vi "_Read_C.vi"(8 "error in (no error)":errorcluster, 11 "Postgres Connector In":refnum<class "Postgres Connector.lvclass">) -> (0 "error out":errorcluster, 1 "Another Query?":bool, 2 "No return?":bool, 3 "Postgres Connector Out":refnum<class "Postgres Connector.lvclass">)   [LabVIEW 2019, in "PG_LIB.lvlib" / "Postgres Connector.lvclass"]
doc: "This VI decode the \"C\" section of the message sent by the database. It also check if a another query has been sent. It return the type of query that has been completed"
uses:
  Postgres Connector.lvclass
  Cluster_Reader_Infos.ctl
  Enum_RowDescription_State_Machine.ctl
  Postgres Connector.lvclass/Postgres Connector.ctl
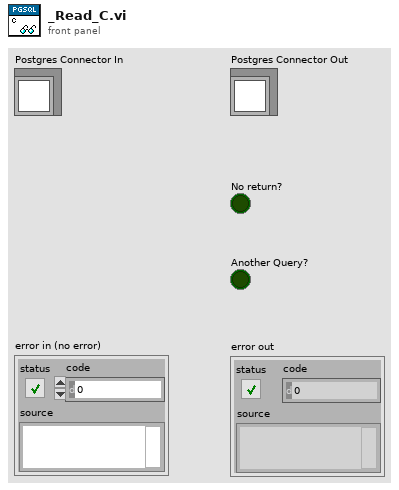
[diagram p1: front panel]
types:
  T1 = typedef "PG_LIB.lvlib/Postgres Connector.lvclass/Cluster_Reader_Infos.ctl" = cluster{"Byte Length":i32}
  T2 = typedef "PG_LIB.lvlib/Postgres Connector.lvclass/Enum_RowDescription_State_Machine.ctl" = enum16{"Check For Error", "Wait For T", "Wait For D", "Wait For Z", "C Byte Length", "Z Byte Length", "n Byte Length", "Byte Length", "Get Infos", "Check For End", "Flush", "Quit"}
  T3 = enum16{"Standard", "Buffered", "CRLF", "Immediate"}
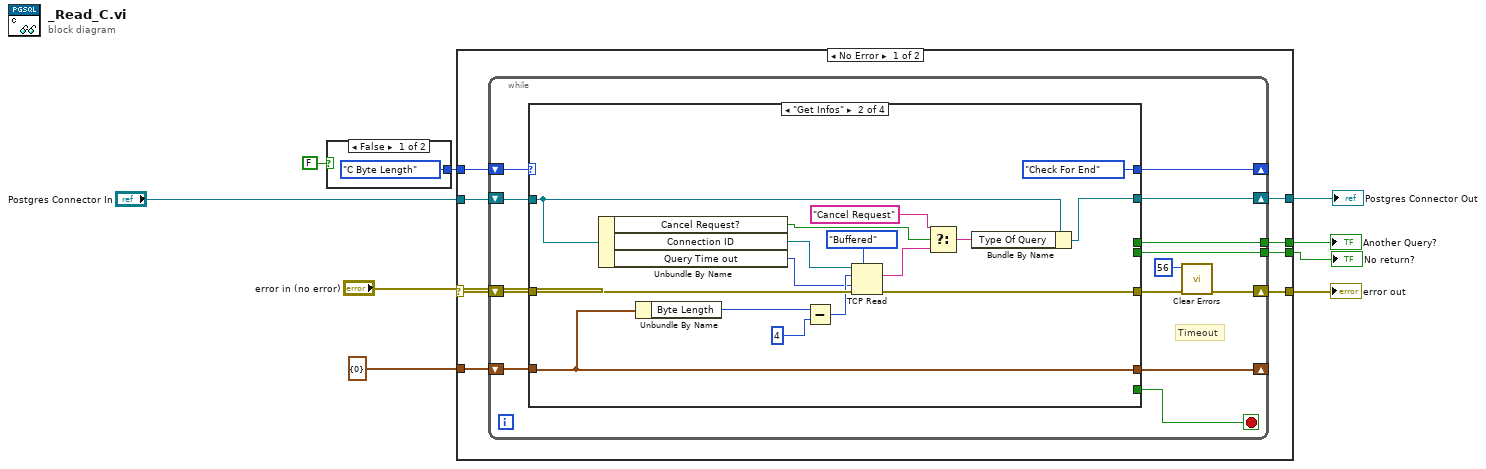
[diagram p0: block diagram]
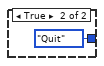
[diagram p2: hidden frame]
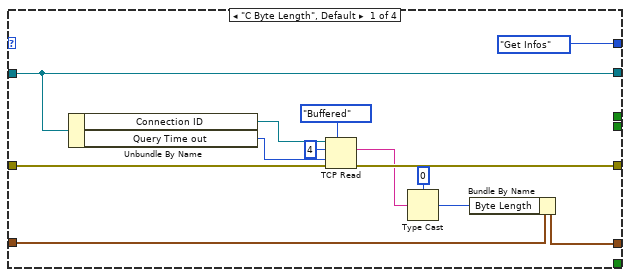
[diagram p3: hidden frame]
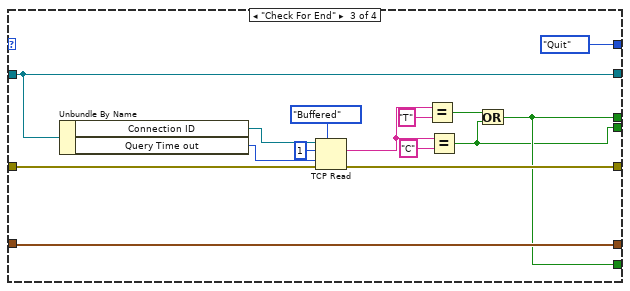
[diagram p4: hidden frame]
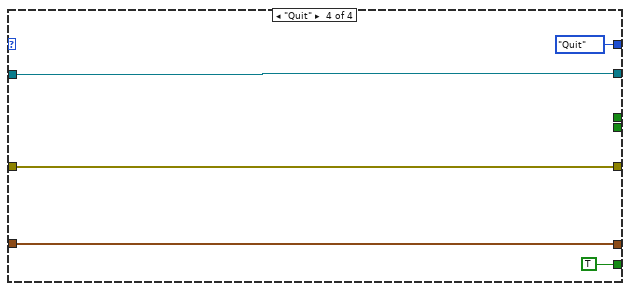
[diagram p5: hidden frame]
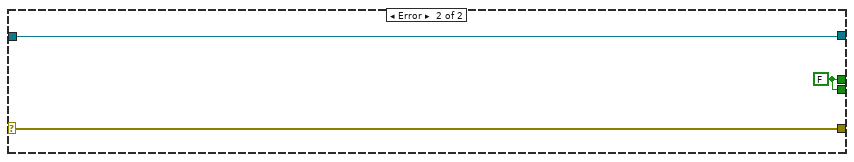
[diagram p6: hidden frame]
diagram:
  n1 = case shown="False" FALSE {
    tunnel: [Enum_RowDescription_State_Machine."C Byte Length" Enum_RowDescription_State_Machine."Quit"] -> w8
    frame False {
    }
    frame True {
    }
  }
  n2 = case shown="No Error" "error in (no error)" {
    selector: "error in (no error)" -> [w18 w84]
    tunnel: "Postgres Connector In" -> [w19 w83]
    tunnel: w8 -> [w17 _]
    tunnel: [w16 w84] -> w7
    tunnel: T1 {"Byte Length"=0} ("Reader_Infos") -> [w15 _]
    tunnel: [w14 w82] -> w5
    tunnel: [w13 w83] -> w4
    tunnel: [w12 w82] -> w3
    frame No Error {
      n3 = while {
        shift-right: [w28] -> w16
        shift-left: w18 -> [w31]
        shift-right: [w26] -> _
        shift-left: w17 -> [w30]
        shift-right: [w24] -> _
        shift-left: w15 -> [w25]
        tunnel: [w22] -> w14
        shift-right: [w21] -> w13
        shift-left: w19 -> [w32]
        tunnel: [w20] -> w12
        stop <- w23 stop-if-true
        # "Timeout"
        n4 = case shown="\"Get Infos\"" w30 {
          tunnel: w32 -> [w41 w52 w68 w77]
          tunnel: w31 -> [w42 w59 w72 w80]
          tunnel: [w40 w58 w71 w80] -> w29
          tunnel: [Enum_RowDescription_State_Machine."Get Infos" Enum_RowDescription_State_Machine."Check For End" Enum_RowDescription_State_Machine."Quit" Enum_RowDescription_State_Machine."Quit"] -> w26
          tunnel: w25 -> [w39 w56 w70 w81]
          tunnel: [w38 w56 w70 w81] -> w24
          tunnel: [_ _ w65 TRUE] -> w23
          tunnel: [_ _ w65 _] -> w22
          tunnel: [w41 w51 w68 w77] -> w21
          tunnel: [_ _ w64 _] -> w20
          frame "C Byte Length", Default {
            n5 = Unbundle By Name(w41) -> ("Connection ID"=w44:refnum<k5>, "Query Time out"=w33:i32)
            n6 = TCP Read(connection ID=w44, bytes to read=4, error in (no error)=w42, 7:T3."Buffered" ("mode (standard)"), 9:w33) -> (data out=w34:string, error out=w40:errorcluster)  [unwired: 1 out]
            n7 = Type Cast(type=0, x=w34) -> (*(type *) &x=w35:i32)
            n8 = Bundle By Name(cluster=w39, "Byte Length"=w35) -> (w38:T1)
          }
          frame "Get Infos" {
            n9 = Unbundle By Name(w52) -> ("Cancel Request?"=w46:bool, "Connection ID"=w60:refnum<k5>, "Query Time out"=w50:i32)
            n10 = Unbundle By Name(w56) -> ("Byte Length"=w55:i32)
            n11 = Subtract(x=w55, y=4 ("bytes to read")) -> (x-y=w54:i32)
            n12 = TCP Read(connection ID=w60, bytes to read=w54, error in (no error)=w59, 7:T3."Buffered" ("mode (standard)"), 9:w50) -> (data out=w49:string, error out=w58:errorcluster)  [unwired: 1 out]
            n13 = Select(t="Cancel Request", s=w46, f=w49) -> (s? t:f=w48:string)
            n14 = Bundle By Name(cluster=w52, "Type Of Query"=w48) -> (w51:refnum<class "Postgres Connector.lvclass">)
          }
          frame "Check For End" {
            n15 = Unbundle By Name(w68) -> ("Connection ID"=w75:refnum<k5>, "Query Time out"=w62:i32)
            n16 = TCP Read(connection ID=w75, bytes to read=1, error in (no error)=w72, 7:T3."Buffered" ("mode (standard)"), 9:w62) -> (data out=w63:string, error out=w71:errorcluster)  [unwired: 1 out]
            n17 = Equal?(x=w63, y="T") -> (x = y?=w66:bool)
            n18 = Equal?(x=w63, y="C") -> (x = y?=w64:bool)
            n19 = Or(x=w66, y=w64) -> (x .or. y?=w65:bool)
          }
          frame "Quit" {
          }
        }
        n20 = call <vilib>:"Clear Errors.vi"("error in (no error)"=w29, "specific error code to clear (0: all)"=56) -> ("error out"=w28:errorcluster)  [unwired: 4 in, 1 out]
      }
    }
    frame Error {
      w82 = FALSE
    }
  }
  "error out" <- w7
  "Another Query?" <- w5
  "Postgres Connector Out" <- w4
  "No return?" <- w3
